vi "BL Disable.vi"(8 "error in (no error)":errorcluster) -> (0 "error out":errorcluster)   [LabVIEW 2019]
uses:
  <instrlib>/niDCPower/nidcpower.llb/niDCPower Wait For Event - Event.ctl
  Globals.vi
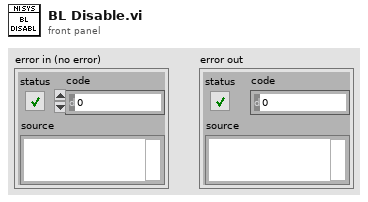
[diagram p1: front panel]
types:
  T1 = typedef "niDCPower Wait For Event - Event.ctl" = i32
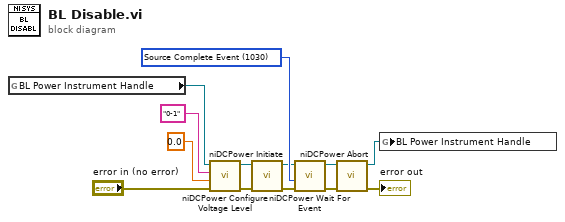
[diagram p0: block diagram]
diagram:
  w9 = T1 1030 items=["Source Complete Event"=1030, "Measure Complete Event"=1031, "Sequence Iteration Complete Event"=1032, "Sequence Engine Done Event"=1033] ("event")
  n1 = global read "Globals.vi" "BL Power Instrument Handle"() -> (w12:refnum<k15>)
  n2 = call <instrlib>:"niDCPower Configure Voltage Level.vi"("error in (no error)"="error in (no error)", "voltage level"=0.0, "channel name"="0-1" ("channels"), "instrument handle"=w12) -> ("error out"=w5:errorcluster, "instrument handle out"=w6:refnum<k15>)  [unwired: 6 out]
  n3 = call <instrlib>:"niDCPower Initiate.vi"("error in (no error)"=w5, "instrument handle"=w6) -> ("error out"=w8:errorcluster, "instrument handle out"=w7:refnum<k15>)  [unwired: 2 in, 6 out]
  n4 = call <instrlib>:"niDCPower Wait For Event.vi"("error in (no error)"=w8, "event"=w9, "instrument handle"=w7) -> ("error out"=w4:errorcluster, "instrument handle out"=w2:refnum<k15>)  [unwired: 1 in, 6 out]
  n5 = call <instrlib>:"niDCPower Abort.vi"("error in (no error)"=w4, "instrument handle"=w2) -> ("error out"=→"error out":errorcluster, "instrument handle out"=w1:refnum<k15>)  [unwired: 8 in]
  n6 = global write "Globals.vi" "BL Power Instrument Handle"(w1) -> ()
